vi "ConvertTo(string).vi"(8 "error in":errorcluster, 9 "Message Payload":variant) -> (0 "error out":errorcluster, 1 "Message Payload string":string)   [LabVIEW 2019]
doc: "Convert variant to string\n\nBolder Software LLC"
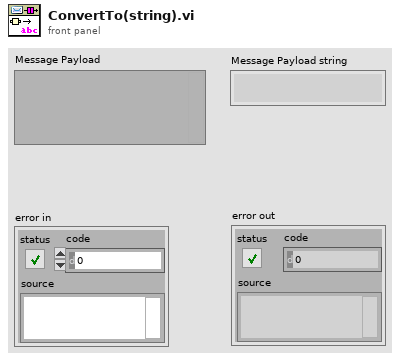
[diagram p1: front panel]
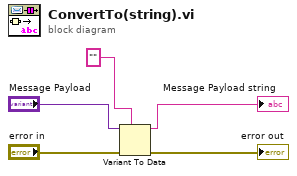
[diagram p0: block diagram]
diagram:
  n1 = Variant To Data(error in="error in", type="" ("Message Payload error"), Variant="Message Payload") -> (data=→"Message Payload string":string, error out=→"error out":errorcluster)
